vi "Write Data.vi"(10 "AO Array":waveform(dbl)[](array[waveform]), 11 "AO Task":refnum<k21>[](array[refnum])) -> ()   [LabVIEW 2013]
uses:
  <vilib>/DAQmx/write.llb/DAQmx Write (Analog 1D Wfm NChan NSamp).vi
  <vilib>/DAQmx/miscellaneous.llb/DAQmx Fill In Error Info.vi
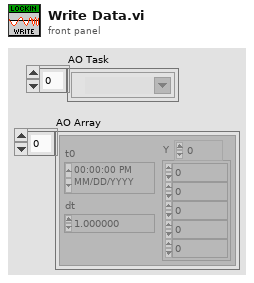
[diagram p1: front panel]
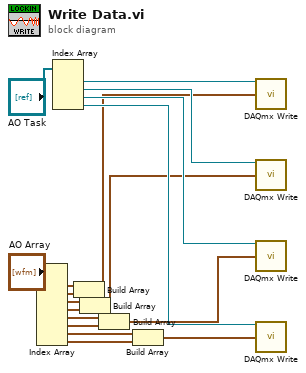
[diagram p0: block diagram]
diagram:
  n1 = Index Array(array="AO Array") -> (element #1=w11:waveform(dbl), element #2=w10:waveform(dbl), element #3=w9:waveform(dbl), element #4=w8:waveform(dbl), element #5=w7:waveform(dbl), element #6=w6:waveform(dbl), element #7=w5:waveform(dbl), element #8=w4:waveform(dbl))  [unwired: 8 in]
  n2 = Index Array(array="AO Task") -> (element #1=w15:refnum<k21>, element #2=w14:refnum<k21>, element #3=w13:refnum<k21>, element #4=w12:refnum<k21>)  [unwired: 4 in]
  n3 = Build Array(w11, w10) -> (w3:waveform(dbl)[])
  n4 = Build Array(w9, w8) -> (w2:waveform(dbl)[])
  n5 = Build Array(w7, w6) -> (w1:waveform(dbl)[])
  n6 = Build Array(w5, w4) -> (w18:waveform(dbl)[])
  n7 = call-poly <vilib>:"DAQmx Write.vi"("task/channels in"=w15, "data"=w3) -> ()  [unwired: 11 in, 3 out]
  n8 = call-poly <vilib>:"DAQmx Write.vi"("task/channels in"=w14, "data"=w2) -> ()  [unwired: 11 in, 3 out]
  n9 = call-poly <vilib>:"DAQmx Write.vi"("task/channels in"=w13, "data"=w1) -> ()  [unwired: 11 in, 3 out]
  n10 = call-poly <vilib>:"DAQmx Write.vi"("task/channels in"=w12, "data"=w18) -> ()  [unwired: 11 in, 3 out]
